vi "do_move.vi"(7 "Absolute":bool, 8 "error in":errorcluster, 9 "Axis positions":dbl[](array[numeric]), 10 "Axis enable":bool[](array[boolean]), 11 "Newmark handle":refnum<visa-resource-name>) -> (0 "error out":errorcluster)   [LabVIEW 2012]
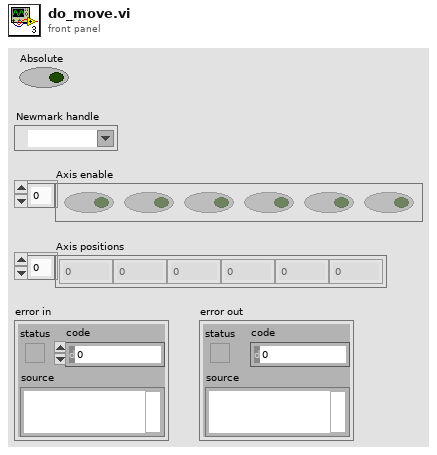
[diagram p1: front panel]
types:
  T1 = typedef "Board Id" = u8
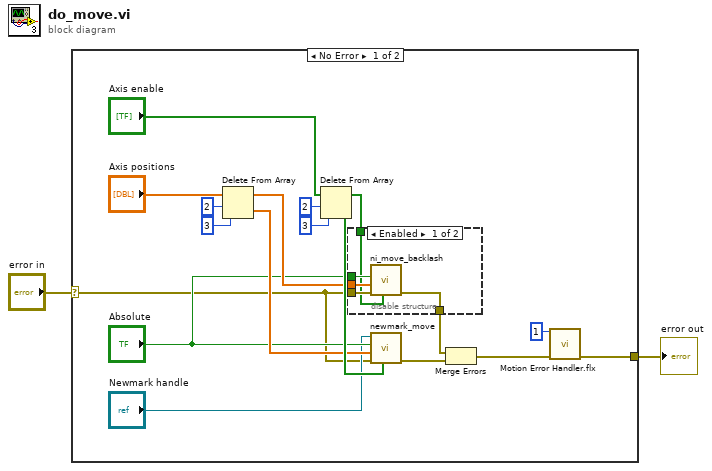
[diagram p0: block diagram]
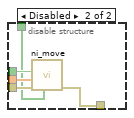
[diagram p2: hidden frame]
diagram:
  n1 = case shown="No Error" "error in" {
    selector: "error in" -> [w3 w31]
    tunnel: [w5 w31] -> w2
    frame No Error {
      n2 = Delete From Array(array="Axis positions", length=2, index=3) -> (deleted portion=w14:dbl[], array with subset deleted=w13:dbl[])
      n3 = Delete From Array(array="Axis enable", length=2, index=3) -> (deleted portion=w18:bool[], array with subset deleted=w17:bool[])
      n4 = disable-structure shown="Enabled" {
        disable-tunnel: "Absolute" -> [w25 w30]
        disable-tunnel: w3 -> [w24 w29]
        disable-tunnel: [w23 w28] -> w9
        disable-tunnel: w13 -> [w22 w27]
        disable-tunnel: w17 -> [w21 w26]
        frame Enabled {
          n5 = call "ni_move_backlash.vi"("Axis enable"=w21, "error in"=w24, "Axis positions"=w22, "Absolute"=w25) -> ("error out"=w23:errorcluster)  [unwired: 7 in]
        }
        frame Disabled {
          n6 = call "ni_move.vi"("Axis enable"=w26, "error in"=w29, "Axis positions"=w27, "Absolute"=w30) -> ("error out"=w28:errorcluster)  [unwired: 7 in]
        }
      }
      n7 = call "newmark_move.vi"("Axis enable"=w18, "error in"=w3, "Axis positions"=w14, "Absolute"="Absolute", "VISA Refnum in"="Newmark handle") -> ("error out"=w10:errorcluster)  [unwired: 4 in, 2 out]
      n8 = Merge Errors(w9, w10) -> (w20:errorcluster)
      n9 = call <vilib>:"Motion Error Handler.flx"("Board ID"=T1 1, "error in (no error)"=w20) -> ("error out"=w5:errorcluster)  [unwired: 9 in, 4 out]
    }
    frame Error {
    }
  }
  "error out" <- w2
